vi "InitializePanels.vi"(8 "error in (no error)":errorcluster, 11 "Maui Manager in":refnum<class "Maui Manager.lvclass">) -> (0 "error out":errorcluster, 3 "Maui Manager out":refnum<class "Maui Manager.lvclass">)   [LabVIEW 2019, in "Maui Manager.lvclass"]
uses:
  Maui Manager.lvclass
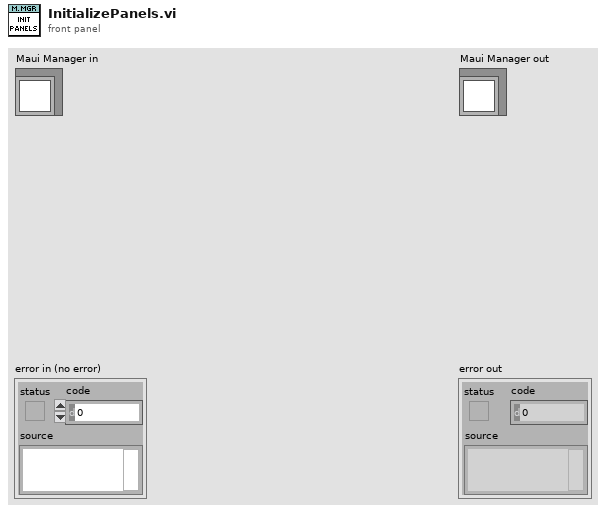
[diagram p1: front panel]
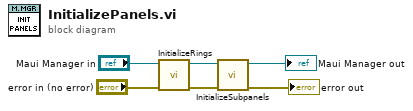
[diagram p0: block diagram]
diagram:
  n1 = call "InitializeRings.vi"("error in (no error)"="error in (no error)", "Maui Manager in"="Maui Manager in") -> ("error out"=w1:errorcluster, "Maui Manager out"=w4:refnum<class "Maui Manager.lvclass">)  [unwired: 8 in]
  n2 = call "InitializeSubpanels.vi"("error in (no error)"=w1, "Maui Manager in"=w4) -> ("error out"=→"error out":errorcluster, "Maui Manager out"=→"Maui Manager out":refnum<class "Maui Manager.lvclass">)  [unwired: 8 in]
